vi "CutImage.vi"(4 "NumPix":dbl, 6 "Size":u8, 7 "PointIn":cluster{"X":dbl, "Y":dbl}, 9 "Width(mm)":dbl, 10 "Angle":dbl, 11 "PyroIn":cluster{"Pyro1":i16[], "X":i16[], "Y":i16[]}) -> (3 "Image":dbl[][](array[numeric]))   [LabVIEW 2014]
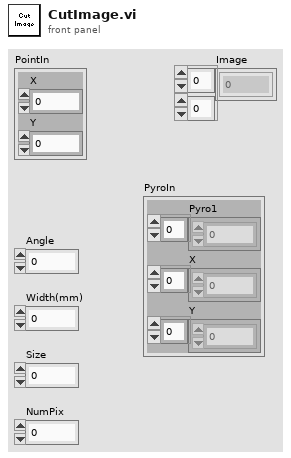
[diagram p1: front panel]
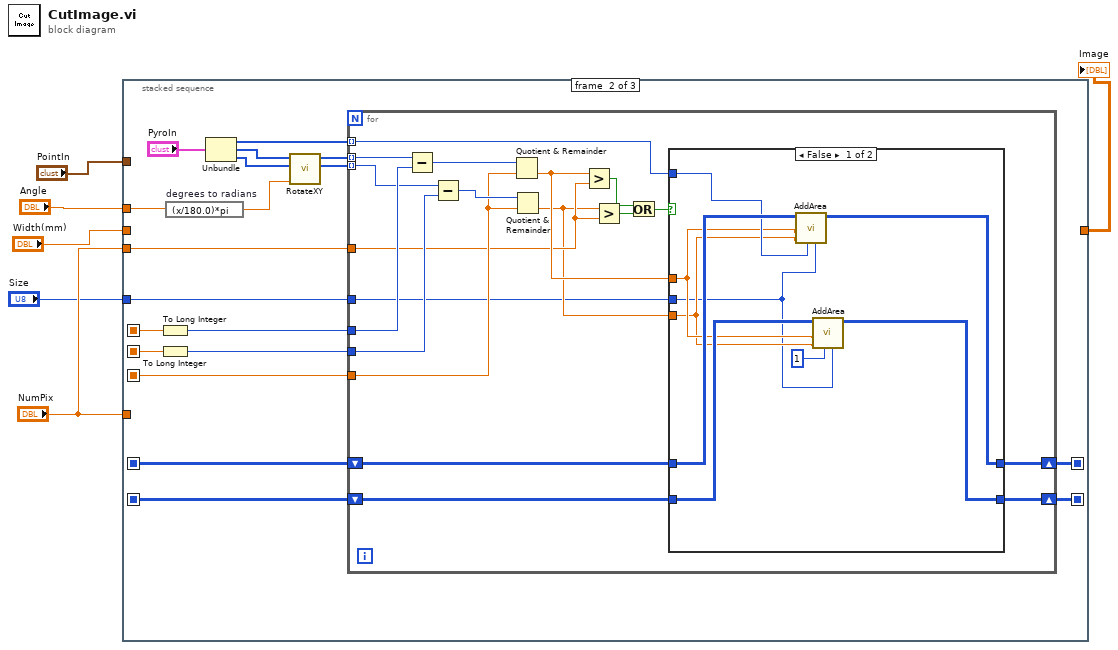
[diagram p0: block diagram]
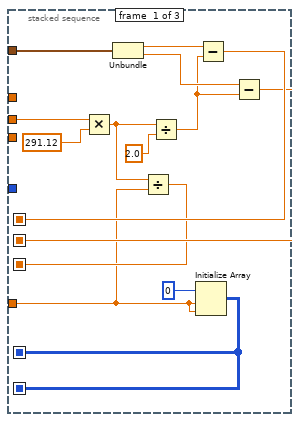
[diagram p2: hidden frame]
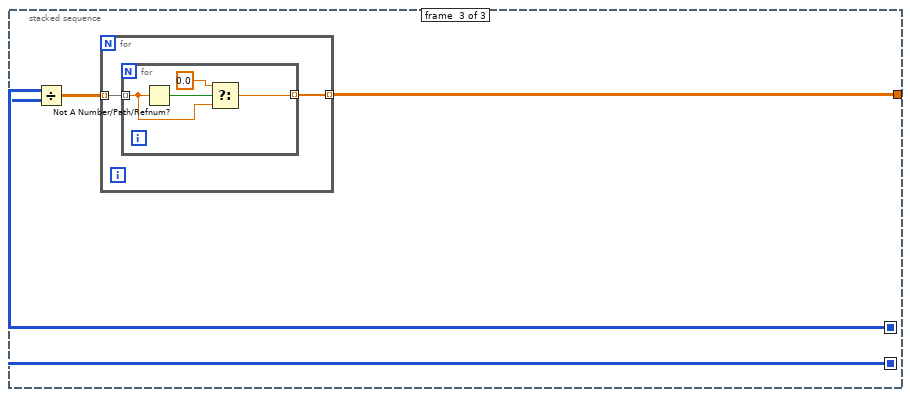
[diagram p4: hidden frame]
diagram:
  n1 = stacked-sequence {
    seq-local: [w15 _ _] -> [_ w39 _]
    seq-local: [w14 _ _] -> [_ w37 _]
    seq-local: [w12 _ _] -> [_ w34 _]
    seq-local: [w12 _ _] -> [_ w33 _]
    seq-local: [w10 _ _] -> [_ w35 _]
    seq-local: [_ w32 _] -> [_ _ w73]
    seq-local: [_ w31 _] -> [_ _ w72]
    tunnel: "Angle" -> [_ w27 _]
    tunnel: "Size" -> [_ w26 _]
    tunnel: "NumPix" -> [_ w25 _]
    tunnel: [_ _ w70] -> w3
    tunnel: "NumPix" -> [w9 _ _]
    tunnel: "Width(mm)" -> [w8 _ _]
    tunnel: "PointIn" -> [w7 _ _]
    frame #0 {
      n2 = Multiply(x=w8, y=291.12) -> (x*y=w11:dbl)
      n3 = Unbundle(w7) -> ("X"=w18:dbl, "Y"=w17:dbl)
      n4 = Divide(x=w11, y=w9) -> (x/y=w10:dbl)
      n5 = Divide(x=w11, y=2.0) -> (x/y=w16:dbl)
      n6 = Initialize Array(u32 0, w9, w9) -> (w12:u32[][])
      n7 = Subtract(x=w18, y=w16) -> (x-y=w15:dbl)
      n8 = Subtract(x=w17, y=w16) -> (x-y=w14:dbl)
    }
    frame #1 {
      n9 = To Long Integer(number=w39) -> (32bit integer=w38:i32)
      n10 = To Long Integer(number=w37) -> (32bit integer=w36:i32)
      n11 = expression code="(x/180.0)*pi" "degrees to radians"(w27) -> (w28:dbl)
      n12 = Unbundle("PyroIn") -> ("Pyro1"=w23:i16[], "X"=w22:i16[], "Y"=w21:i16[])
      n13 = call "RotateXY.vi"("Angle"=w28, "Y"=w21, "X"=w22) -> ("Yout"=w29:i16[], "Xout"=w30:i16[])  [unwired: 7 in]
      n14 = for {
        tunnel: w30 -> [w58] mode=indexing
        tunnel: w29 -> [w56] mode=indexing
        tunnel: w23 -> [w50] mode=indexing
        tunnel: w38 -> [w57]
        tunnel: w36 -> [w55]
        tunnel: w35 -> [w44]
        tunnel: w25 -> [w42]
        shift-right: [w49] -> w32
        shift-left: w34 -> [w51]
        shift-right: [w47] -> w31
        shift-left: w33 -> [w48]
        tunnel: w26 -> [w40]
        n15 = Subtract(x=w58, y=w57) -> (x-y=w45:i32)
        n16 = Subtract(x=w56, y=w55) -> (x-y=w46:i32)
        n17 = Quotient & Remainder(x=w45, y=w44) -> (floor(x/y)=w43:dbl)  [unwired: 1 out]
        n18 = Quotient & Remainder(x=w46, y=w44) -> (floor(x/y)=w41:dbl)  [unwired: 1 out]
        n19 = Greater?(x=w43, y=w42) -> (0:w54:bool)
        n20 = Greater?(x=w41, y=w42) -> (0:w53:bool)
        n21 = Or(x=w54, y=w53) -> (x .or. y?=w52:bool)
        n22 = case shown="False" w52 {
          tunnel: w51 -> [w67 w69]
          tunnel: w43 -> [w62 _]
          tunnel: w41 -> [w61 _]
          tunnel: w50 -> [w65 _]
          tunnel: [w66 w69] -> w49
          tunnel: w48 -> [w64 w68]
          tunnel: [w63 w68] -> w47
          tunnel: w40 -> [w59 _]
          frame False {
            n23 = call "AddArea.vi"("Size"=w59, "Value"=w65, "Yloc"=w61, "Xloc"=w62, "ArrayIn"=w67) -> ("ArrayOut"=w66:u32[][])  [unwired: 6 in]
            n24 = call "AddArea.vi"("Size"=w59, "Value"=u32 1, "Yloc"=w61, "Xloc"=w62, "ArrayIn"=w64) -> ("ArrayOut"=w63:u32[][])  [unwired: 6 in]
          }
          frame True {
          }
        }
      }
    }
    frame #2 {
      n25 = Divide(x=w73, y=w72) -> (x/y=w71:dbl[][])
      n26 = for {
        tunnel: w71 -> [w75] mode=indexing
        tunnel: [w74] -> w70 mode=indexing
        n27 = for {
          tunnel: w75 -> [w78] mode=indexing
          tunnel: [w76] -> w74 mode=indexing
          n28 = Not A Number/Path/Refnum?(number/path/refnum=w78) -> (NaN/Path/Refnum?=w79:bool)
          n29 = Select(t=0.0, s=w79, f=w78) -> (s? t:f=w76:dbl)
        }
      }
    }
  }
  "Image" <- w3
